vi "Stop Core.vi"(10 "final error code":i32, 11 "Nested in":refnum<class "UI_Top_Customer.lvclass">) -> (3 "Nested out":refnum<class "UI_Top_Customer.lvclass">)   [LabVIEW 2021, in "UI_Top_Customer.lvclass"]
doc: "(<B>Filename</B>: Actor Framework.lvlib:Actor.lvclass:Stop Core.vi)\n\nDefines what the actor does before it stops. Use the <B>final error code</B> input to determine whether the actor shut down in response to an error.\n\nBy default, this method does nothing. A descendant class may override it to define behavior, such as shutting down any processes the actor initiated in its override of the Actor Core method."
uses:
  UI_Top_Customer.lvclass
  <userlib>/John_Lib/AbstractActorTemplate/AbstractActorTemplate/UIActorTop.lvclass
  UI_Top_Customer.lvclass/UI_Top_Customer.ctl
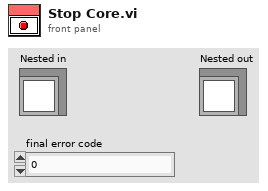
[diagram p1: front panel]
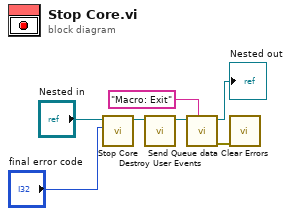
[diagram p0: block diagram]
diagram:
  n1 = call-parent "Stop Core.vi"("final error code"="final error code", "Nested in"="Nested in") -> ("Nested out"=w5:refnum<class "UI_Top_Customer.lvclass">)  [unwired: 9 in]
  n2 = call "Destroy User Events.vi"("UI Template in"=w5) -> ("UI Template out"=w3:refnum<class "UI_Top_Customer.lvclass">)  [unwired: 10 in]
  n3 = call "Send Queue data.vi"("Elements in Front"="Macro: Exit", "UI_Top_Customer in"=w3) -> ("error out"=w1:errorcluster, "UI_Top_Customer out"=→"Nested out":refnum<class "UI_Top_Customer.lvclass">)  [unwired: 8 in]
  n4 = call <vilib>:"Clear Errors.vi"("error in (no error)"=w1) -> ()  [unwired: 5 in, 2 out]
